vi "Get Image from Ref.vi"(8 "error in (no error)":errorcluster, 11 "Class Reference Control in":refnum<class "Class Reference Control.lvclass">) -> (0 "error out":errorcluster, 2 "new picture":picture, 3 "Class Reference Control out":refnum<class "Class Reference Control.lvclass">)   [LabVIEW 2016, in "Class Reference Control.lvclass"]
uses:
  Class Reference Control.lvclass
  Class Reference Control.lvclass/Class Reference Control.ctl
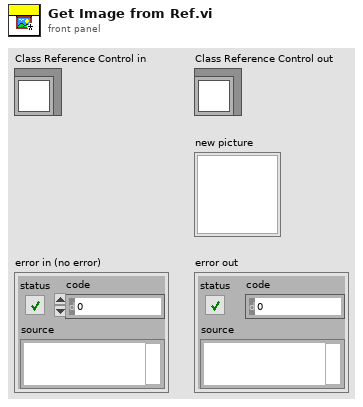
[diagram p1: front panel]
types:
  T1 = typedef "imagedata.ctl" = cluster{"image type":i32, "image depth":i32, "image":u8[], "mask":u8[], "colors":u32[], "Rectangle":cluster{"left":i16, "top":i16, "right":i16, "bottom":i16}}
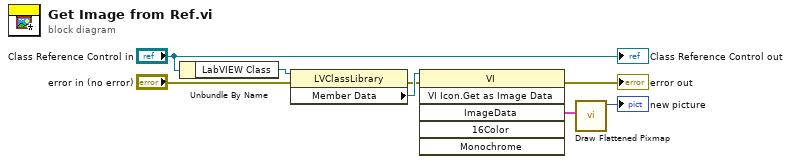
[diagram p0: block diagram]
diagram:
  n1 = Unbundle By Name("Class Reference Control in") -> ("LabVIEW Class"=w7:refnum<vi>)
  n2 = property class="LVClassLibrary"(reference=w7, error in="error in (no error)") -> (error out=w2:errorcluster, "Member Data"=w5:refnum<vi>)  [unwired: 1 out]
  n3 = invoke class="VI" method="VI Icon.Get as Image Data"(reference=w5, error in=w2) -> (error out=→"error out":errorcluster, "ImageData"=w6:T1)  [unwired: 4 in, 4 out]
  n4 = call <vilib>:"Draw Flattened Pixmap.vi"("image data"=w6) -> ("new picture"=→"new picture":picture)  [unwired: 8 in]
  "Class Reference Control out" <- "Class Reference Control in"
